vi "Create Workspace Ring Channel.vi"(8 "error in (no error)":errorcluster, 10 "Enum":variant, 11 "Channel Ref in":T1 format="%.0x") -> (0 "error out":errorcluster, 3 "Channel Ref out":T1 format="%.0x")   [LabVIEW 2019, in "FPGA Addon System Explorer.lvlib"]
uses:
  FPGA Addon System Explorer.lvlib
  <vilib>/NI VeriStand/Custom Device API/Custom Device Item Ref.ctl
  <vilib>/NI VeriStand/Custom Device API/Custom Device API.lvlib
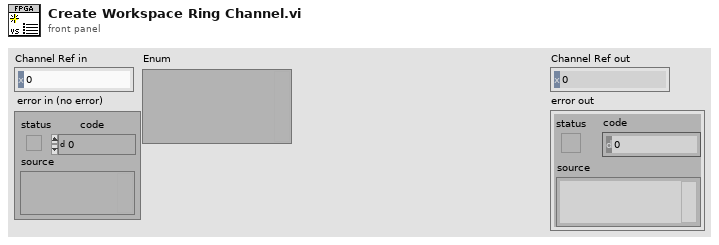
[diagram p1: front panel]
types:
  T1 = typedef "Custom Device API.lvlib/Custom Device Item Ref.ctl" = u64
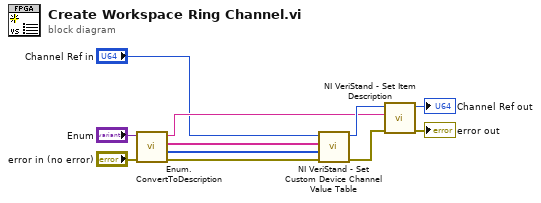
[diagram p0: block diagram]
diagram:
  n1 = call "Enum.ConvertToDescription.vi"("error in (no error)"="error in (no error)", "Enum"="Enum") -> ("error out"=w6:errorcluster, "Number"=w10:i32[], "Values"=w11:string[], "Description"=w8:string)  [unwired: 6 in]
  n2 = call <vilib>:"NI VeriStand - Set Custom Device Channel Value Table.vi"("error in (no error)"=w6, "Values"=w10, "Names"=w11, "Channel Ref in"="Channel Ref in") -> ("error out"=w7:errorcluster, "Channel Ref out"=w9:T1)  [unwired: 6 in]
  n3 = call <vilib>:"NI VeriStand - Set Item Description.vi"("error in (no error)"=w7, "Description"=w8, "Item Ref in"=w9) -> ("error out"=→"error out":errorcluster, "Item Ref out"=→"Channel Ref out":T1)  [unwired: 6 in, 1 out]
